vi "Measure.vi"(0 "Yokogawa WT500 in":refnum<class "Yokogawa WT500.lvclass">, 1 "Card Number":u8=1 min=1 step=1, 5 "Measurement Type":T1, 7 "Preset (2: Preset 2)":u16(ring)=2 items=["", "Preset1", "Preset2", "Preset3", "Preset4"], 9 "Number of Item (255)":i32=255 min=1 max=255 step=1, 11 "error in (no error)":errorcluster) -> (4 "Yokogawa WT500 out":refnum<class "Yokogawa WT500.lvclass">, 8 "Array":dbl[](array[numeric]), 15 "error out":errorcluster)   [LabVIEW 2012]
uses:
  Universal Power Meter class/Master Control.ctl
  Universal Power Meter class/Universal Power Meter.lvclass
  Yokogawa WT500.lvclass
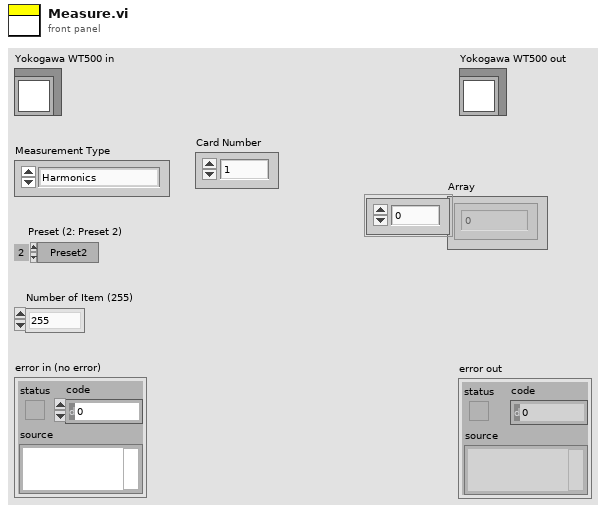
[diagram p1: front panel]
types:
  T1 = typedef "Universal Power Meter.lvlib/Universal Power Meter.lvclass/Master Control.ctl" = enum16{"Harmonics", "RMS"}
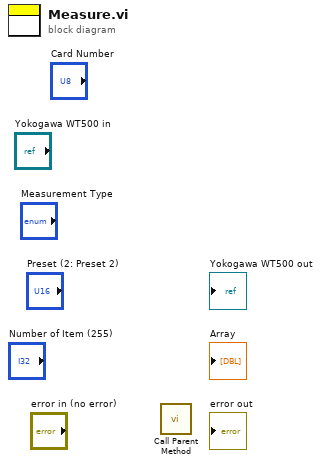
[diagram p0: block diagram]
diagram:
  n1 = call-parent "Call Parent Method"() -> ()  [unwired: 7 in, 3 out]
